vi "Test XML Write.vi"() -> ()   [LabVIEW 2015]
uses:
  Data.ctl
panel:
  in  "Data In":T1 {"Time" format="%<%H:%M:%S%2u>T"}
  out "resulting string":string
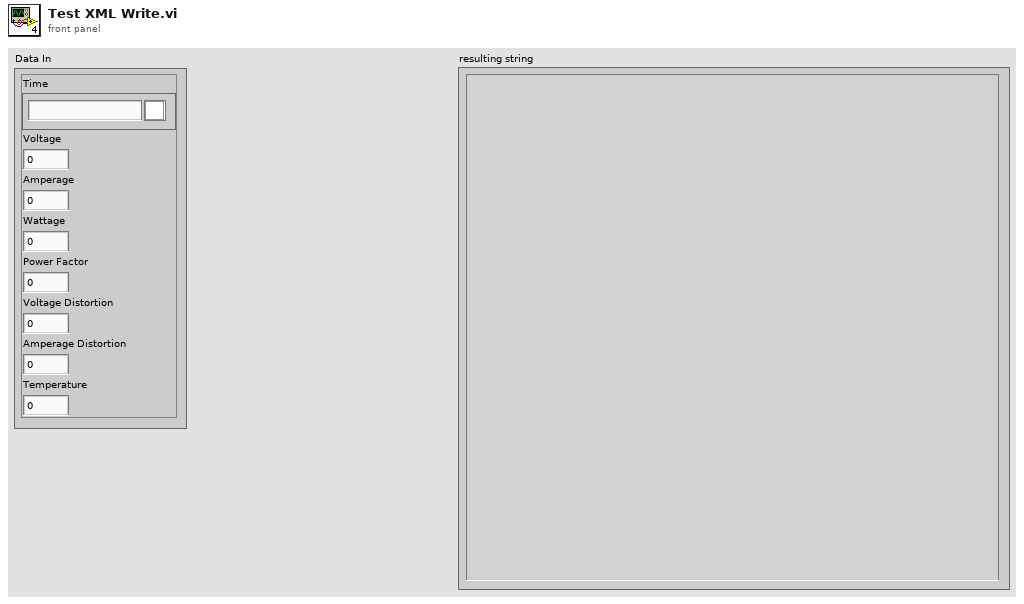
[diagram p1: front panel]
types:
  T1 = typedef "Data.ctl" = cluster{"Time":timestamp, "Voltage":dbl, "Amperage":dbl, "Wattage":dbl, "Power Factor":dbl, "Voltage Distortion":dbl, "Amperage Distortion":dbl, "Temperature":dbl}
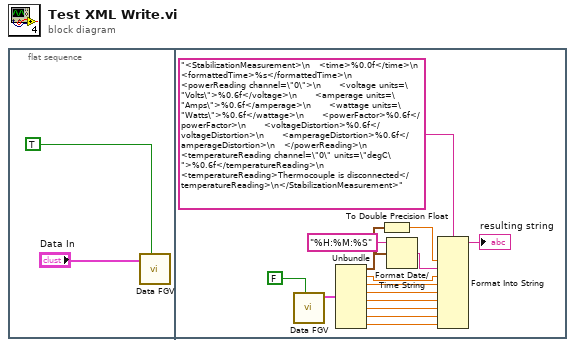
[diagram p0: block diagram]
diagram:
  n1 = flat-sequence {
    frame #0 {
      n2 = call "Data FGV.vi"("Write?"=TRUE, "Data In"="Data In") -> ()  [unwired: 9 in, 1 out]
    }
    frame #1 {
      n3 = call "Data FGV.vi"("Write?"=FALSE) -> ("Data Out"=w4:T1)  [unwired: 10 in]
      n4 = Unbundle(w4) -> ("Time"=w15:timestamp, "Voltage"=w7:dbl, "Amperage"=w8:dbl, "Wattage"=w9:dbl, "Power Factor"=w10:dbl, "Voltage Distortion"=w11:dbl, "Amperage Distortion"=w12:dbl, "Temperature"=w14:dbl)
      n5 = To Double Precision Float(number=w15) -> (double precision float=w6:dbl)
      n6 = Format Date/Time String(time format string (%c)="%H:%M:%S", seconds (now)=w15) -> (date/time string=w16:string)  [unwired: 1 in]
      n7 = Format Into String(format string="<StabilizationMeasurement>\n   <time>%0.0f</time>\n   <formattedTime>%s</formattedTime>\n   <powerReading channel=\"0\">\n      <voltage units=\"Volts\">%0.6f</voltage>\n      <amperage units=\"Amps\">%0.6f</amperage>\n      <wattage units=\"Watts\">%0.6f</wattage>\n      <powerFactor>%0.6f</powerFactor>\n      <voltageDistortion>%0.6f</voltageDistortion>\n      <amperageDistortion>%0.6f</amperageDistortion>\n   </powerReading>\n   <temperatureReading channel=\"0\" units=\"degC\">%0.6f</temperatureReading>\n   <temperatureReading>Thermocouple is disconnected</temperatureReading>\n</StabilizationMeasurement>", w6, w16, w7, w8, w9, w10, w11, w12, w14) -> (resulting string=→"resulting string":string)  [unwired: 2 in, 1 out]
    }
  }
